vi "uA_daq_Set_uA_mA_Current_Range.vi"(8 "error in":errorcluster, 9 "Opamp Current Range - Branch 1 & 2":T1(ring), 11 "device name":tag="Dev4") -> (0 "error out":errorcluster)   [LabVIEW 2015]
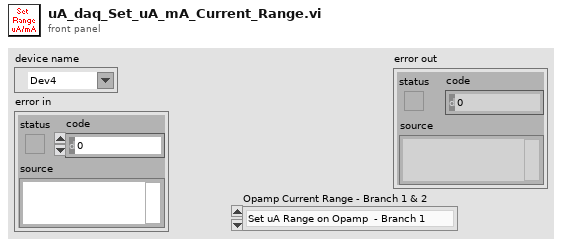
[diagram p1: front panel]
types:
  T1 = enum16{"Set uA Range on Opamp  - Branch 1", "Set mA Range on Opamp - Branch 2"}
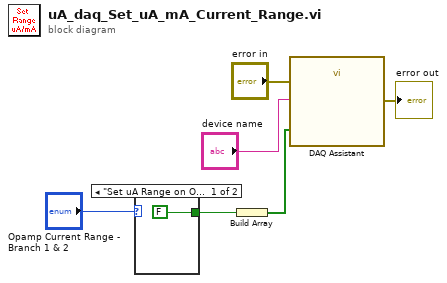
[diagram p0: block diagram]
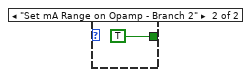
[diagram p2: hidden frame]
diagram:
  n1 = case shown="\"Set uA Range on Opamp  - Branch 1\", Default" "Opamp Current Range - Branch 1 & 2" {
    tunnel: [FALSE TRUE] -> w5
    frame "Set uA Range on Opamp  - Branch 1", Default {
    }
    frame "Set mA Range on Opamp - Branch 2" {
    }
  }
  n2 = Build Array(w5) -> (w4:bool[])
  n3 = call "DAQ Assistant"("data"=w4, "error in"="error in", "device name"="device name") -> ("error out"=→"error out":errorcluster)  [unwired: 15 in, 1 out]
